vi "LQR_no_integrator.vi"() -> ()   [LabVIEW 2021]
uses:
  <vilib>/Simulation/Scripting/Companion Diagram/SimConfigNode/SimParams.ctl
  <vilib>/Simulation/Scripting/Companion Diagram/SimConfigNode/_simSolvers.ctl
  <vilib>/Simulation/Implementation/Shared/SIMSCR Execution Mode.ctl
  <vilib>/Simulation/Param Hierarchy/Typedefs/SIMPH Param Control Actions.ctl
  <vilib>/Simulation/Implementation/Shared/SIM limit type.ctl
  <vilib>/Simulation/Implementation/Shared/NILVSim_ParamChanged.vi
  <vilib>/Simulation/Implementation/Shared/NILVSIM_BeginStep.vi
  <vilib>/Simulation/DataSources/Implementation/NILVSim Step.llb/SIM Step (scalar).vi
  <vilib>/Simulation/ContinuousLinear/Implementation/NILVSim Integrator new.llb/SIM Integrator Distributor (vector).vi
  <vilib>/Simulation/SignalArithmetic/Implementation/NILVSim Gain.llb/SIM Gain (vector,ScalarGain).vi
  <vilib>/Simulation/ContinuousLinear/Implementation/NILVSim State Space.llb/SIM State Space Distributor (CD).vi
  <vilib>/Simulation/SignalDisplay/Implementation/NILVSim Time Waveform.llb/SIM Time Waveform (vector).vi
  <vilib>/Simulation/SignalArithmetic/Implementation/NILVSim Gain.llb/SIM Gain (vector,MatrixGain).vi
  <vilib>/Simulation/ContinuousLinear/Implementation/NILVSim State Space.llb/SIM State Space Collector (CD).vi
  <vilib>/Simulation/ContinuousLinear/Implementation/NILVSim Integrator new.llb/SIM Integrator Collector (vector).vi
  <vilib>/Simulation/Implementation/Shared/NILVSim_Manager.vi
  <vilib>/Utility/error.llb/Clear Errors.vi
  <vilib>/Simulation/Implementation/Shared/NILVSim_FinalizeModel.vi
  <vilib>/addons/Control Design/_Model Construction/Model Creation.llb/Model Creation SubVI/cd_Create State Space Model.vi
  <vilib>/addons/Control Design/_Dynamic Analysis/Dynamic Analysis.llb/Dynamic Analysis subVI/cd_Poles (State-Space).vi
  <vilib>/addons/Control Design/_Dynamic Analysis/Dynamic Analysis.llb/Dynamic Analysis subVI/cd_Pole-Zero Map (State-Space).vi
  <vilib>/addons/Control Design/_Utility/Model Viewer.llb/Model Viewer SubVI/cd_Draw State-Space Equation (SS).vi
  <vilib>/addons/Control Design/_State Feedback Control/State Feedback Control.llb/State Feedback Control SubVis/cd_Linear Quadratic Regulator.vi
  <vilib>/Simulation/Implementation/Shared/SIM Unbundle Sim Info.vi
  <vilib>/Simulation/Implementation/Shared/NILVSim_Initialize.vi
  <vilib>/Simulation/Utility/Implementation/NILVSim Get Time and IsAcceptedStep.vi
  <vilib>/Simulation/Implementation/Shared/SIMSH Read Queue.vi
  <vilib>/Simulation/Implementation/Shared/NILVSim_GetModelError.vi
  <vilib>/Simulation/Implementation/Shared/SIM Bundle Sim Info.vi
  <vilib>/Simulation/Scripting/Companion Diagram/SimConfigNode/SimDog.xnode
  <vilib>/Simulation/Implementation/XNodeFramework/SimXNode/SimX.xnode
  <vilib>/addons/Control Design/_Model Construction/NI_LinSys_Model Creation.lvlib
  <vilib>/addons/Control Design/_State-Space Analysis/NI_CD_State-Space Analysis.lvlib
  <vilib>/addons/Control Design/_Utility/NI_CD_Model Viewer.lvlib
  <vilib>/addons/Control Design/_Dynamic Analysis/NI_CD_Dynamic Analysis.lvlib
  <vilib>/addons/Control Design/_Model Construction/Model Typedefs.llb/CD General Elements.ctl
  <vilib>/addons/Control Design/_Model Construction/NI_LinSys_Model Typedefs.lvlib
  <vilib>/addons/Control Design/_Model Construction/Model Typedefs.llb/CD State Space Model (MIMO).ctl
  <vilib>/Simulation/ContinuousLinear/Implementation/NILVSim State Space.llb/SIM State Space (CD).vi
  <vilib>/Simulation/ContinuousLinear/Implementation/NILVSim Integrator new.llb/SIM Integrator (vector).vi
  <vilib>/addons/Control Design/_State Feedback Control/NI_CD_State Feedback Control.lvlib
  <vilib>/Simulation/Implementation/Shared/NI_SIM_Implementation.lvlib
panel:
  out "open loop Poles":cdb[](array[numeric])=[31.622776601683793+0.0i, -31.622776601683793+0.0i, 0.0+0.0i] format="%.3f"
  out "open loop Poles with error stete":cdb[](array[numeric])=[31.622776601683793+0.0i, -31.622776601683793+0.0i, 0.0+0.0i] format="%.3f"
  out "Ki":dbl=100.00000000000021
  out "K":dbl[][](array[numeric])=[[-228.36422016500336, -32.33686509284722]]
  out "control action u":waveform(dbl)[](graph)=[{"t0"=timestamp(10 s since 1904-01-01), "dt"=1.0, "Y"=[99.99619127950126]}]
  out "states":waveform(dbl)[](graph)=[{"t0"=timestamp(10 s since 1904-01-01), "dt"=1.0, "Y"=[0.999961862460632]}, {"t0"=timestamp(10 s since 1904-01-01), "dt"=1.0, "Y"=[4.0542821168364276e-05]}]
  out "Riccati Solution (X)":dbl[][](array[numeric])=[[4140.896470224251, 22.836422016500336, -3233.686509284723], [22.836422016500336, 3.233686509284722, -10.000000000000021], [-3233.686509284723, -10.000000000000021, 12836.422016500315]] format="%.2f"
  in  "Weighting Type":T1(ring)
  in  "R":dbl[][](array[numeric])=[[1.0]] format="%.2f"
  in  "Q":dbl[][](array[numeric])=[[10.0, 0.0, 0.0], [0.0, 1000.0, 0.0], [0.0, 0.0, 10000.0]] format="%.2f"
  out "size(s)":i32[](array[numeric])=[1, 3]
  in  "refernce":dbl=1.0
  out "state y measured":waveform(dbl)[](graph)=[{"t0"=timestamp(10 s since 1904-01-01), "dt"=1.0, "Y"=[0.999961862460632]}]
  out "System":cluster{dbl[], dbl[]}[](graph)=[{[31.622776601683793, -31.622776601683793, 0.0], [0.0, 0.0, 0.0]}, {[-0.0], [0.0]}]
  out "Gain":dbl[][](array[numeric])=[[-228.36422016500336, -32.33686509284722, 100.00000000000021]] format="%.2f"
  out "State  Space Model":picture
  out "Transformed Model":picture
  in  "Form Type":u16(ring)=2 items=["Modal"=0, "Companion"=5, "Controllability"=1, "Controller Companion"=2, "Observability"=3, "Observer Companion"=4]
  out "Transformation Matrix (T)":dbl[][](array[numeric])=[[0.0, -0.1, 0.0], [-0.1, 0.0, 0.0], [0.0, 0.0, 0.1]] format="%.2f"
  out "Is Controllable?":bool=TRUE
  out "Controllability Matrix":dbl[][](array[numeric])=[[0.0, -10.0, 0.0], [-10.0, 0.0, -10000.0], [0.0, 0.0, 10.0]] format="%.2f"
  in  "D":dbl[][](array[numeric]) format="%#.5g"
  in  "C":dbl[][](array[numeric])=[[1.0, 0.0, 0.0]] format="%#.5g"
  in  "B":dbl[][](array[numeric])=[[0.0], [-10.0], [0.0]] format="%#.5g"
  in  "A":dbl[][](array[numeric])=[[0.0, 1.0, 0.0], [1000.0, 0.0, 0.0], [-1.0, 0.0, 0.0]] format="%#.5g"
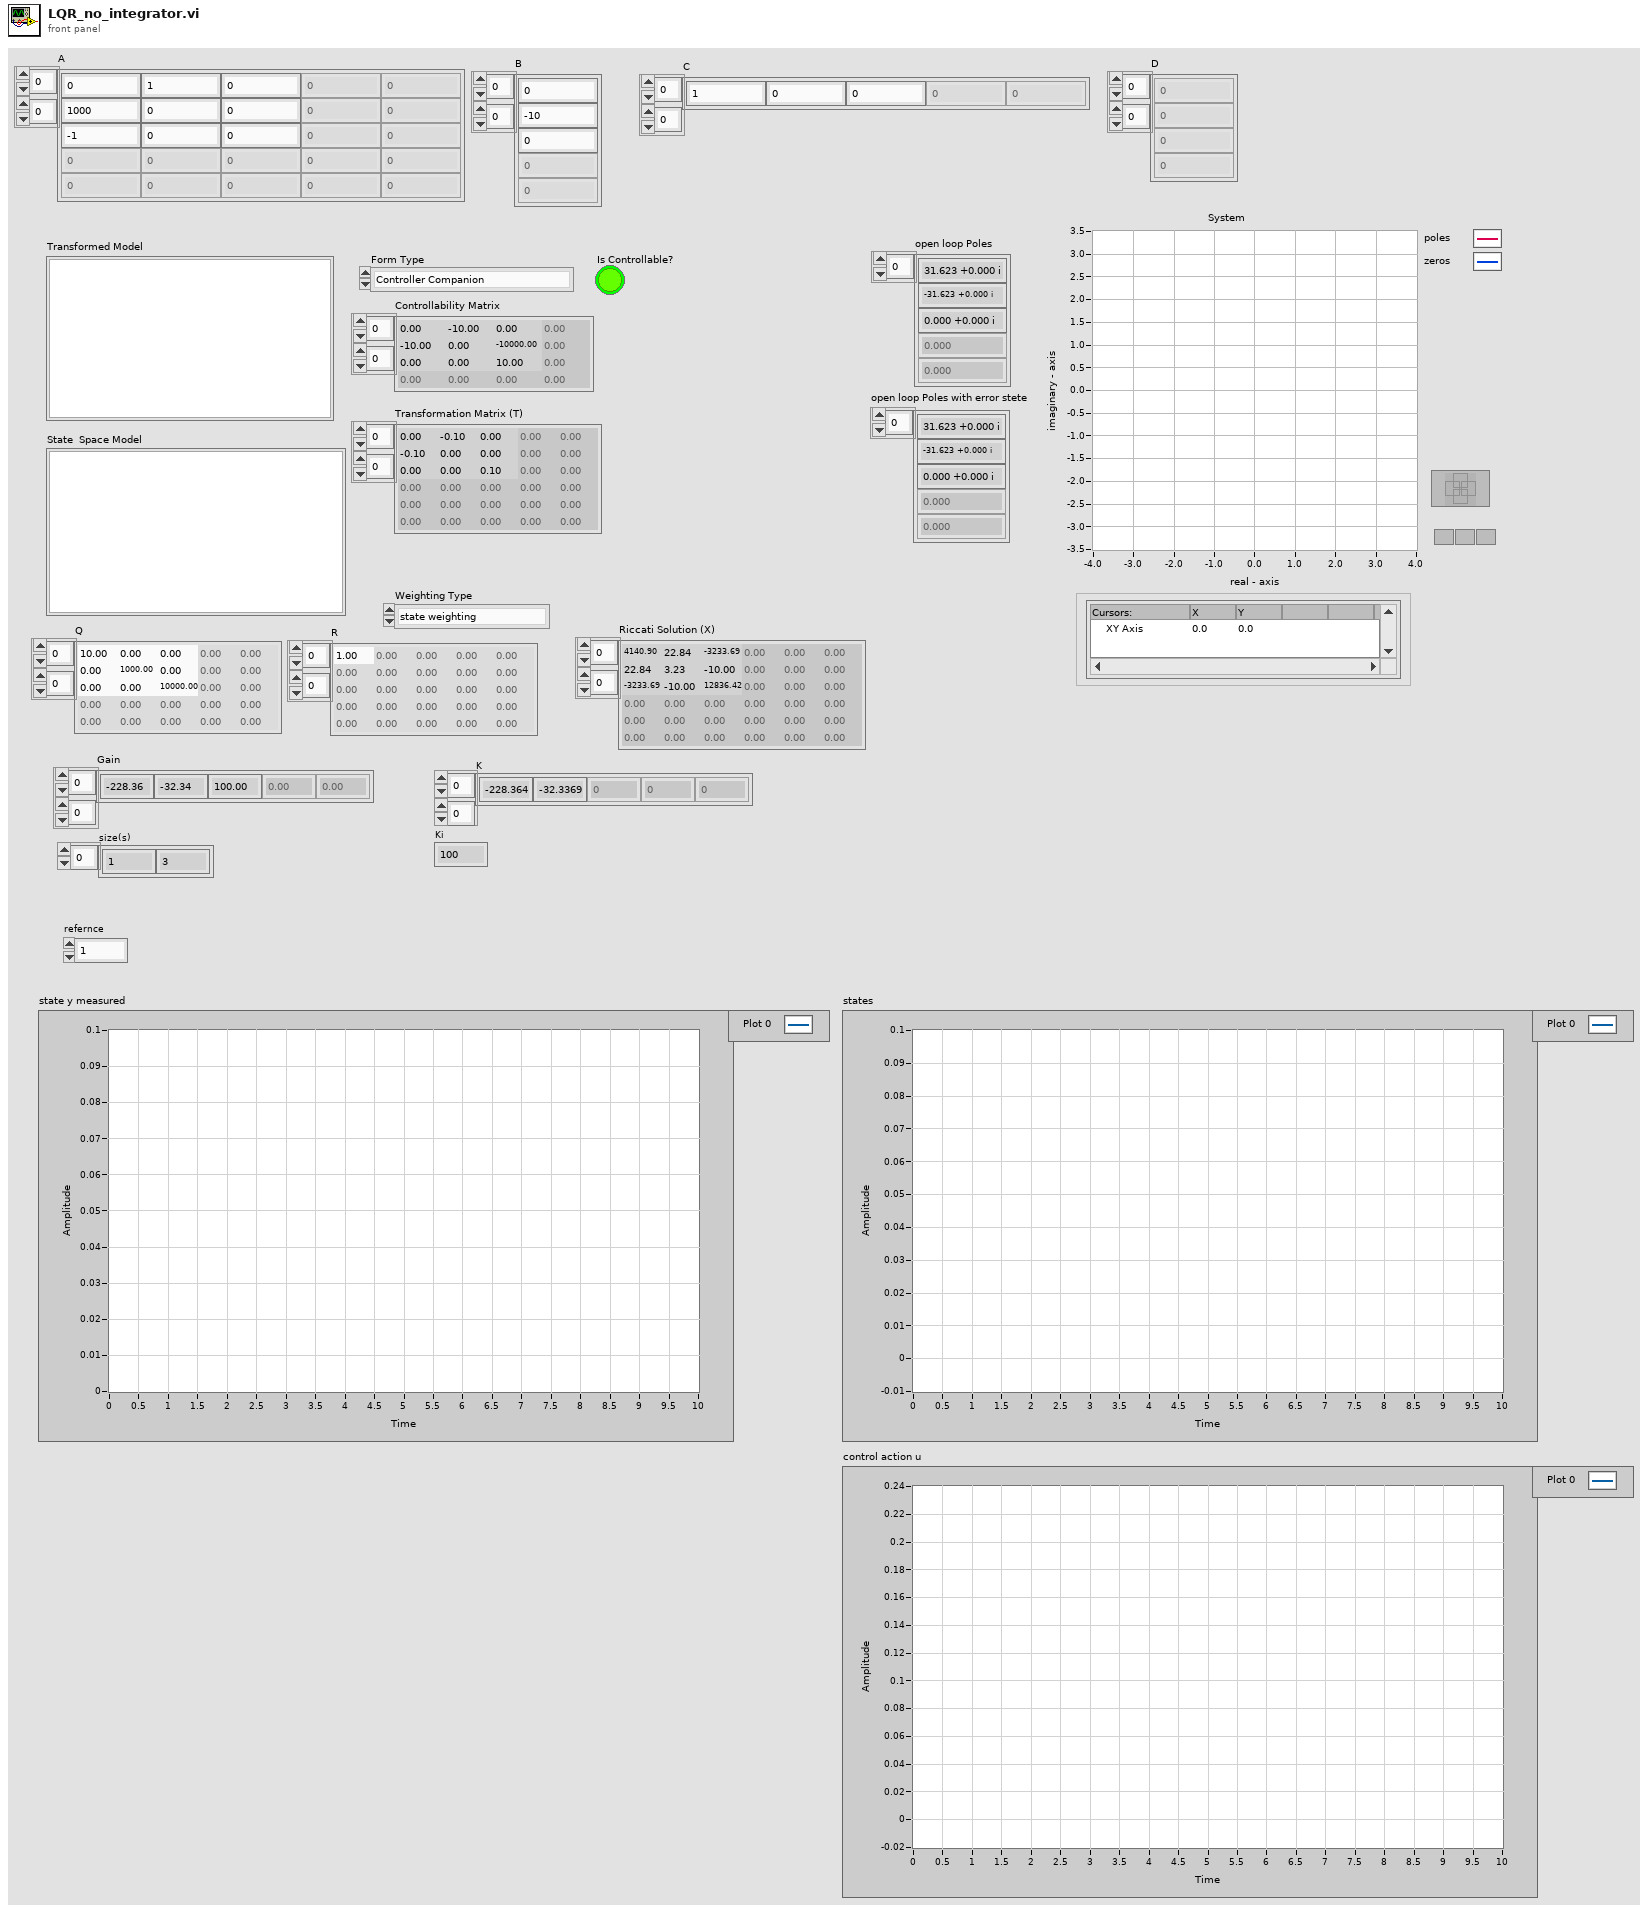
[diagram p1: front panel]
types:
  T1 = enum16{"state weighting", "output weighting, Dim Q = Ny", "output weighting, Dim Q = Nx"}
  T2 = typedef "NI_LinSys_Model Typedefs.lvlib/CD State Space Model (MIMO).ctl" = cluster{"properties":T3, "A":dbl[][], "B":dbl[][], "C":dbl[][], "D":dbl[][], "StateNames":string[], "Transport Delay":dbl[][]}
  T3 = typedef "NI_LinSys_Model Typedefs.lvlib/CD General Elements.ctl" = cluster{"Model name":string, "Input names":string[], "Output names":string[], "Input Delays":dbl[], "Output Delays":dbl[], "Sampling Time":dbl, "Notes":string}
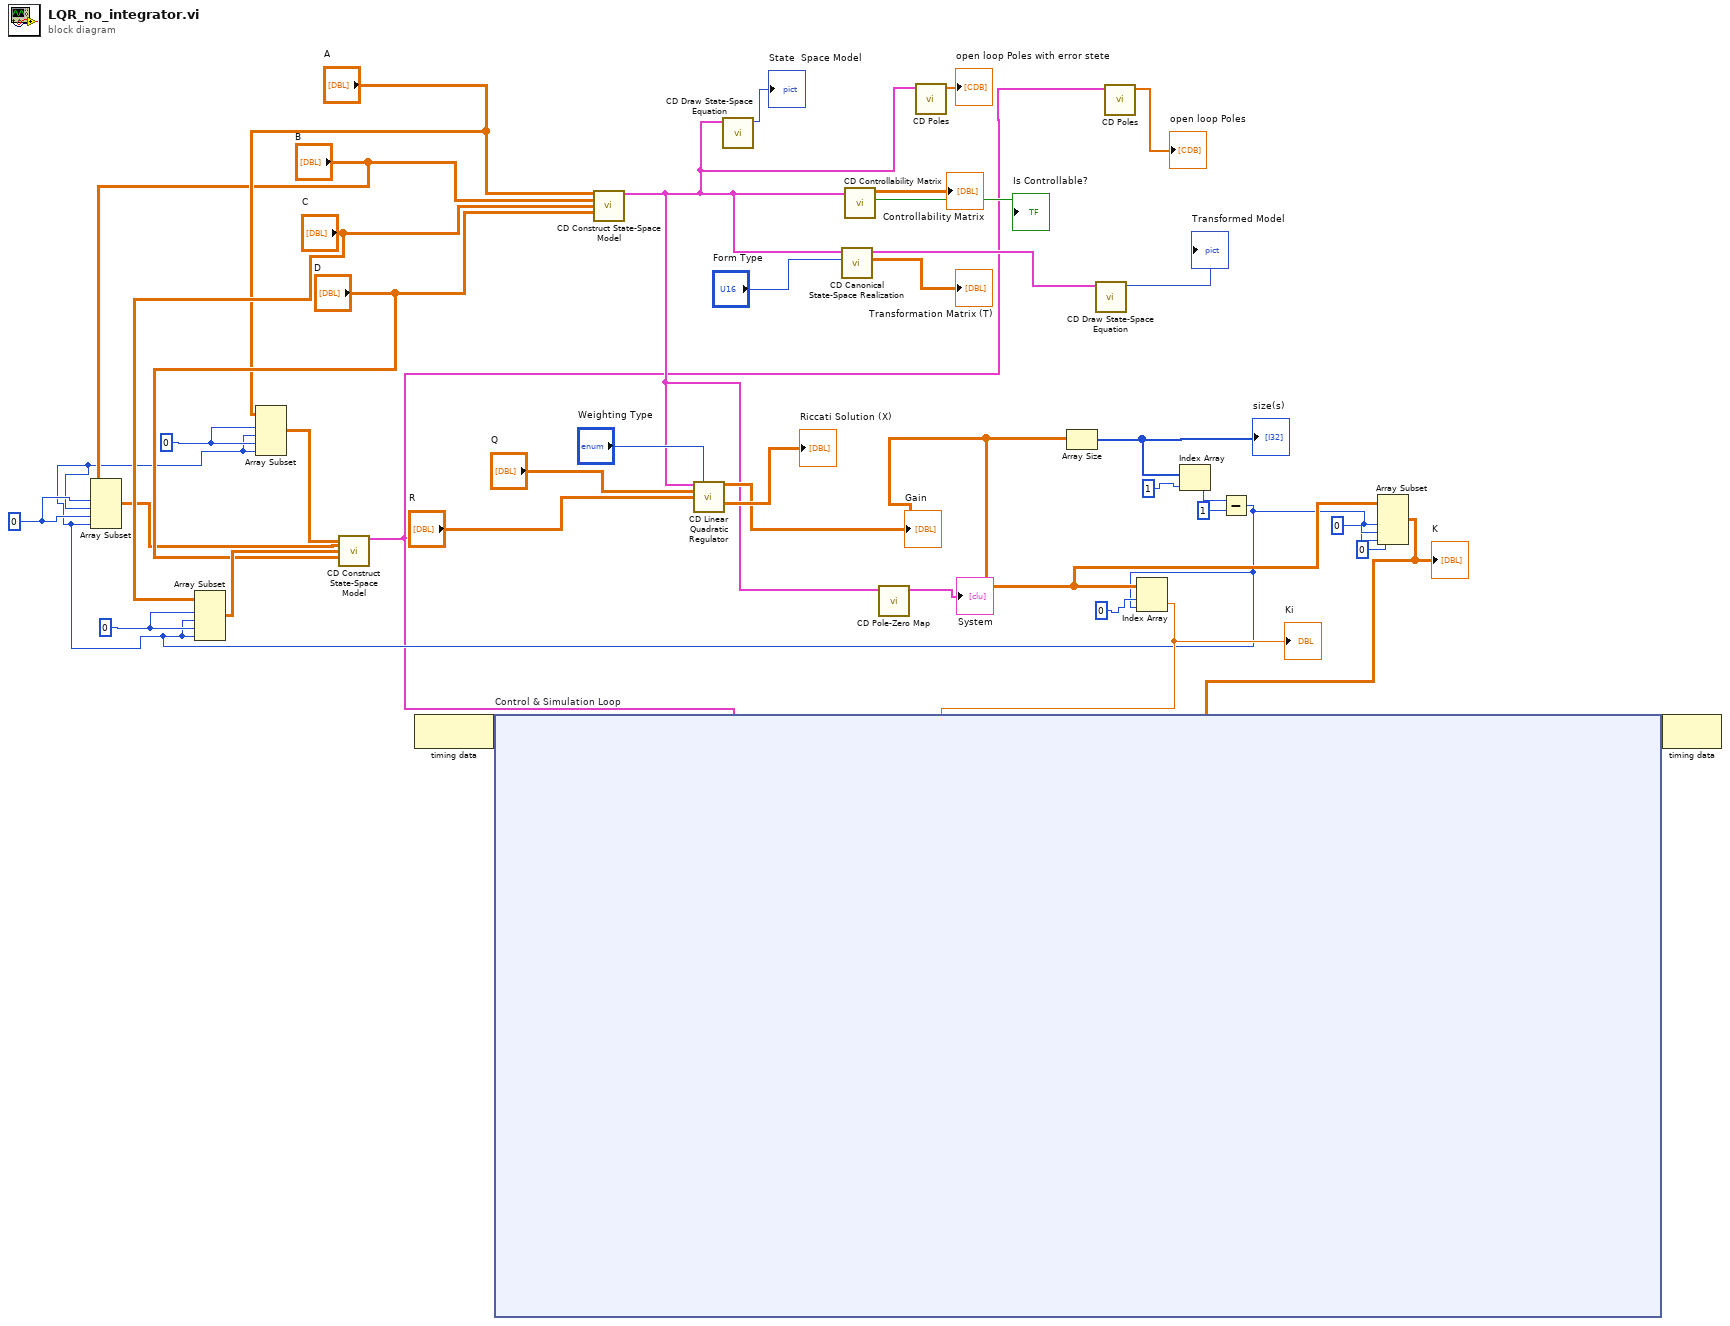
[diagram p0: block diagram]
diagram:
  w16 = 0 ("index")
  w17 = 0 ("index")
  w19 = 0 ("index")
  n1 = node-c288() -> (w31:variant)  [unwired: 1 in]
  n2 = call-poly <vilib>:"CD Construct State-Space Model.vi"("A"="A", "B"="B", "C"="C", "D"="D") -> ("State-Space Model"=w2:T2)  [unwired: 10 in, 1 out]
  n3 = call-poly <vilib>:"CD Linear Quadratic Regulator.vi"("State-Space Model"=w2, "Weighting Type"="Weighting Type", "Q"="Q", "R"="R") -> ("Optimal Gain (K)"=w7:dbl[][], "Riccati Solution (X)"=→"Riccati Solution (X)":dbl[][])  [unwired: 8 in, 2 out]
  "Gain" <- w7
  n4 = call-poly <vilib>:"CD Draw State-Space Equation.vi"("State-Space Model"=w2) -> ("Equation"=→"State  Space Model":picture)  [unwired: 8 in, 2 out]
  n5 = call <vilib>:"CD Canonical State-Space Realization.vi"("Form Type"="Form Type", "State-Space Model"=w2) -> ("Transformation Matrix (T)"=→"Transformation Matrix (T)":dbl[][], "Transformed Model"=w34:T2)  [unwired: 7 in, 1 out]
  n6 = call <vilib>:"CD Controllability Matrix.vi"("State-Space Model"=w2) -> ("Is Controllable?"=→"Is Controllable?":bool, "Controllability Matrix"=→"Controllability Matrix":dbl[][])  [unwired: 7 in, 2 out]
  n7 = call-poly <vilib>:"CD Pole-Zero Map.vi"("State-Space Model"=w2) -> ("Pole-Zero Map"=→"System":cluster{dbl[], dbl[]}[])  [unwired: 7 in, 3 out]
  n8 = call-poly <vilib>:"CD Poles.vi"("State-Space Model"=w2) -> ("Poles"=→"open loop Poles with error stete":cdb[])  [unwired: 9 in, 1 out]
  n9 = Array Size(array=w7) -> (size(s)=w28:i32[])
  "size(s)" <- w28
  n10 = call-poly <vilib>:"CD Draw State-Space Equation.vi"("State-Space Model"=w34) -> ("Equation"=→"Transformed Model":picture)  [unwired: 8 in, 2 out]
  n11 = Index Array(array=w28, index=1 ("index (row)")) -> (element=w27:i32)
  n12 = Subtract(x=w27, y=1) -> (x-y=w6:i32)
  n13 = Array Subset(array="B", index (row)=w17, length (row)=w6, index (col)=w17, length (col)=w6) -> (w12:dbl[][])
  n14 = Array Subset(array="C", index (row)=w16, length (row)=w6, index (col)=w16, length (col)=w6) -> (w15:dbl[][])
  n15 = Array Subset "Array Subset"(array="A", index (row)=w19, length (row)=w6, index (col)=w19, length (col)=w6) -> (w18:dbl[][])
  n16 = call-poly <vilib>:"CD Construct State-Space Model.vi"("A"=w18, "B"=w12, "C"=w15, "D"="D") -> ("State-Space Model"=w1:T2)  [unwired: 10 in, 1 out]
  n17 = call-poly <vilib>:"CD Poles.vi"("State-Space Model"=w1) -> ("Poles"=→"open loop Poles":cdb[])  [unwired: 9 in, 1 out]
  n18 = Index Array(array=w7, index (row)=0, index (col)=w6) -> (element=w25:dbl)
  "Ki" <- w25
  n19 = Array Subset(array=w7, index (row)=0 ("index"), length (row)=w6, index (col)=0 ("index"), length (col)=w6) -> (w5:dbl[][])
  "K" <- w5
  n20 = node-c254 "Control & Simulation Loop"(w31, w1, w25, w5) -> (w30:variant)
  n21 = node-c288(w30) -> ()  [unwired: 1 out]
